vi "Main Base.vi"() -> ()   [LabVIEW 2021]
uses:
  Class Selector.ctl
  Key class/Key.lvclass
  C:/Users/javix/Downloads/Fatory Pattern/Format Key Class/Format Key Class.lvclass
  csv/csv.lvclass
  Format Key Class/Format Key Class.lvclass
  Library.lvlib
panel:
  in  "Class":T1
  out "Value":string
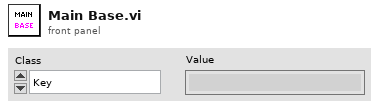
[diagram p1: front panel]
types:
  T1 = typedef "Library.lvlib/Class Selector.ctl" = enum16{"Key", "CSV"}
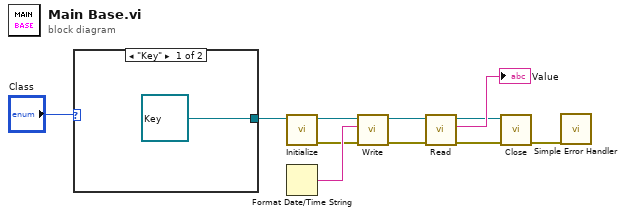
[diagram p0: block diagram]
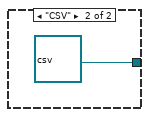
[diagram p2: hidden frame]
diagram:
  n1 = case shown="\"Key\"" "Class" {
    tunnel: [refnum<class "Key.lvclass"> refnum ("Library.lvlib:Key") refnum<class "csv.lvclass"> refnum ("Library.lvlib:csv.lvclass")] -> w1
    frame "Key" {
    }
    frame "CSV" {
    }
  }
  n2 = call-dynamic "Initialize.vi"("Format Key Class in"=w1) -> ("error out"=w4:errorcluster, "Format Key Class out"=w3:refnum<class "Format Key Class.lvclass">)  [unwired: 9 in]
  n3 = Format Date/Time String() -> (date/time string=w10:string)  [unwired: 3 in]
  n4 = call-dynamic "Write.vi"("error in (no error)"=w4, "Value"=w10, "Format Key Class in"=w3) -> ("error out"=w6:errorcluster, "Format Key Class out"=w5:refnum<class "Format Key Class.lvclass">)  [unwired: 7 in]
  n5 = call-dynamic "Read.vi"("error in (no error)"=w6, "Format Key Class in"=w5) -> ("error out"=w8:errorcluster, "Value"=→"Value":string, "Format Key Class out"=w7:refnum<class "Format Key Class.lvclass">)  [unwired: 7 in]
  n6 = call-dynamic "Close.vi"("error in (no error)"=w8, "Format Key Class in"=w7) -> ("error out"=w9:errorcluster)  [unwired: 8 in, 1 out]
  n7 = call <vilib>:"Simple Error Handler.vi"("error in (no error)"=w9) -> ()  [unwired: 4 in, 5 out]
